vi "get_stopThread.vi"(0 "HGF_ThreadWorker":refnum<class "HGF_ThreadWorker.lvclass">, 5 "error in (no error)":errorcluster) -> (14 "dup HGF_ThreadWorker":refnum<class "HGF_ThreadWorker.lvclass">, 16 "stopThread":bool, 19 "error out":errorcluster)   [LabVIEW 2014, in "HGF_BaseClasses.lvlib" / "HGF_ThreadWorker.lvclass"]
doc: "read the stopThread flag and the stop occurence"
uses:
  HGF_ThreadWorker.lvclass
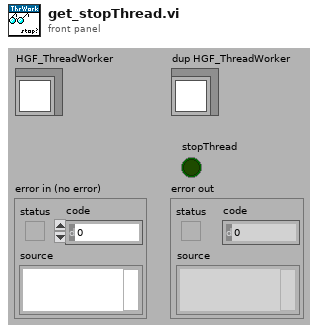
[diagram p1: front panel]
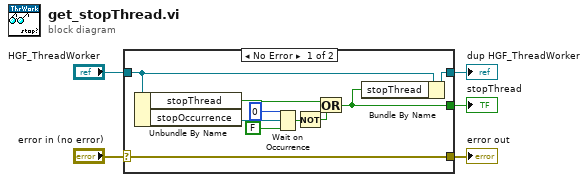
[diagram p0: block diagram]
diagram:
  n1 = case shown="No Error" "error in (no error)" {
    selector: "error in (no error)" -> [w15 w16]
    tunnel: [w15 w16] -> w4
    tunnel: [w7 w17] -> w2
    tunnel: "HGF_ThreadWorker" -> [w14 w17]
    tunnel: [w6 _] -> w1
    frame No Error {
      n2 = Unbundle By Name(w14) -> ("stopThread"=w9:bool, "stopOccurrence"=w10:refnum<k4>)
      n3 = Wait on Occurrence(1:FALSE ("ignore previous (T)"), 2:w10, 3:0 ("ms timeout (-1)")) -> (0:w12:bool)
      n4 = Not(x=w12) -> (.not. x?=w8:bool)
      n5 = Or(x=w9, y=w8) -> (x .or. y?=w6:bool)
      n6 = Bundle By Name(cluster=w14, "stopThread"=w6) -> (w7:refnum<class "HGF_ThreadWorker.lvclass">)
    }
    frame Error {
    }
  }
  "error out" <- w4
  "dup HGF_ThreadWorker" <- w2
  "stopThread" <- w1
